vi "Update Test Server.vi"() -> ()   [LabVIEW 2013, in "OPC UA tests.lvlib"]
doc: "Forces the server to update every line in given input."
uses:
  OPC UA tests.lvlib
  <vilib>/opcua/NI OPC UA Server.lvlib
  <vilib>/OPCUA/server/Write Bool.vi
  module/configuration/OPC UA Data Type.ctl
  module/configuration/OPC UA configuration.lvclass
panel:
  out "error out":errorcluster
  in  "error in (no error)":errorcluster
  in  "OPC UA server refnum in":refnum<k21>
  in  "Items":cluster{"name":string, "OPC UA Data Type":T1}[](array[cluster])
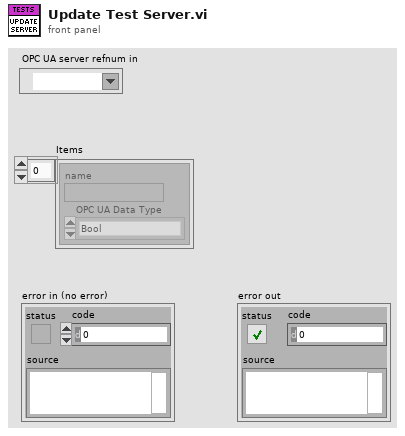
[diagram p1: front panel]
types:
  T1 = typedef "OPC UA configuration.lvclass/OPC UA Data Type.ctl" = enum16{"Bool", "SByte", "Byte", "Int16", "UInt16", "Int32", "UInt32", "Int64", "UInt64", "Float", "Double", "String", "DateTime", "ByteString", "Bool Array", "SByte Array", "Byte Array", "Int16 Array", "UInt16 Array", "Int32 Array", "UInt32 Array", "Int64 Array", "UInt64 Array", "Float Array", "Double Array", "String Array", "DateTime Array", "ByteString Array"}
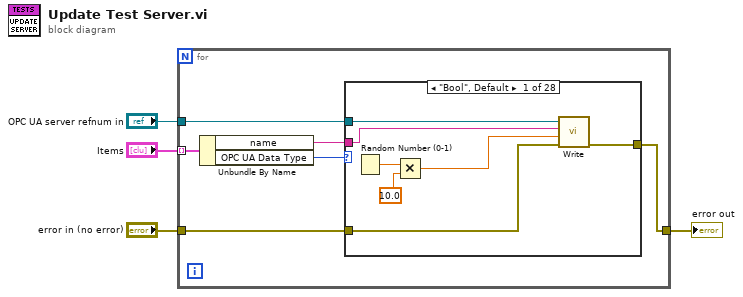
[diagram p0: block diagram]
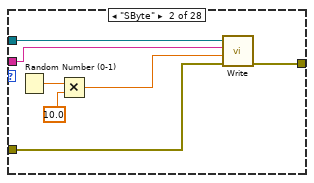
[diagram p2: hidden frame]
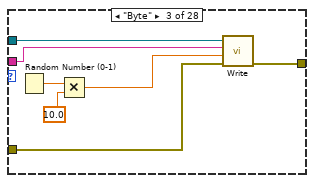
[diagram p3: hidden frame]
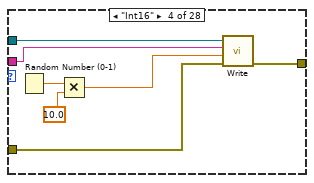
[diagram p4: hidden frame]
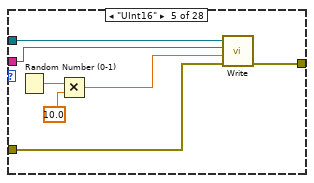
[diagram p5: hidden frame]
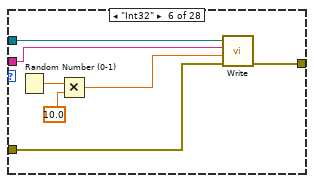
[diagram p6: hidden frame]
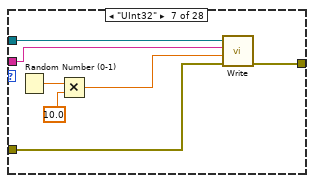
[diagram p7: hidden frame]
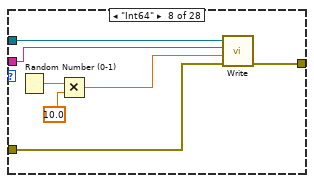
[diagram p8: hidden frame]
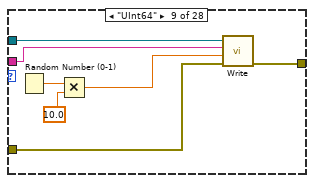
[diagram p9: hidden frame]
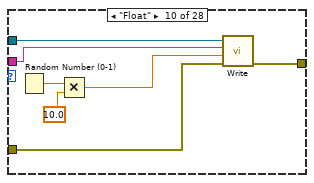
[diagram p10: hidden frame]
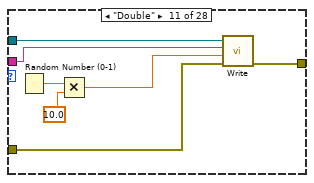
[diagram p11: hidden frame]
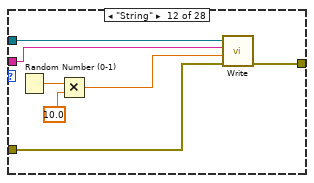
[diagram p12: hidden frame]
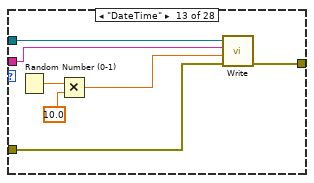
[diagram p13: hidden frame]
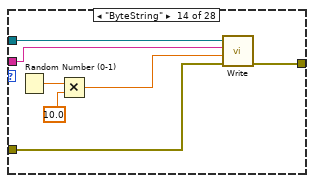
[diagram p14: hidden frame]
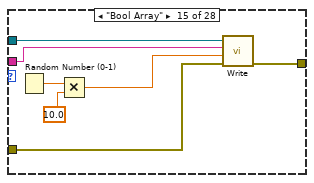
[diagram p15: hidden frame]
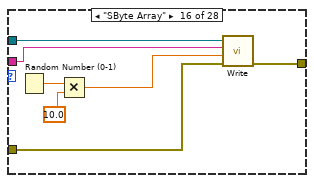
[diagram p16: hidden frame]
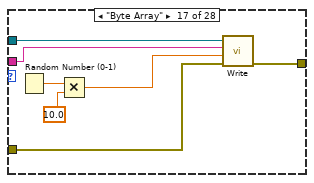
[diagram p17: hidden frame]
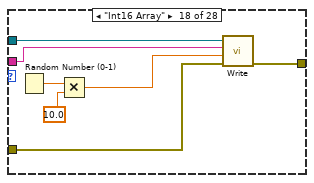
[diagram p18: hidden frame]
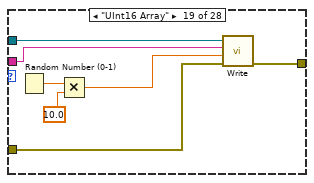
[diagram p19: hidden frame]
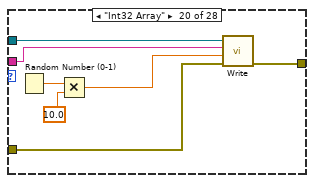
[diagram p20: hidden frame]
diagram:
  n1 = for {
    tunnel: "OPC UA server refnum in" -> [w10]
    tunnel: "Items" -> [w9] mode=indexing
    tunnel: "error in (no error)" -> [w6]
    tunnel: [w5] -> w1
    n2 = Unbundle By Name(w9) -> ("name"=w7:string, "OPC UA Data Type"=w8:T1)
    n3 = case shown="\"Bool\", Default" w8 {
      tunnel: w10 -> [w17 w24 w31 w38 w45 w52 w59 w66 w73 w80 w87 w94 w101 w108 w115 w122 w129 w136 w143 w150 w157 w164 w171 w178 w185 w192 w199 w206]
      tunnel: w7 -> [w16 w23 w30 w37 w44 w51 w58 w65 w72 w79 w86 w93 w100 w107 w114 w121 w128 w135 w142 w149 w156 w163 w170 w177 w184 w191 w198 w205]
      tunnel: w6 -> [w15 w22 w29 w36 w43 w50 w57 w64 w71 w78 w85 w92 w99 w106 w113 w120 w127 w134 w141 w148 w155 w162 w169 w176 w183 w190 w197 w204]
      tunnel: [w14 w21 w28 w35 w42 w49 w56 w63 w70 w77 w84 w91 w98 w105 w112 w119 w126 w133 w140 w147 w154 w161 w168 w175 w182 w189 w196 w203] -> w5
      frame "Bool", Default {
        n4 = Random Number (0-1)() -> (number: 0 to 1=w13:dbl)
        n5 = Multiply(x=w13, y=10.0) -> (x*y=w11:dbl)
        n6 = call-poly <vilib>:"Write.vi"("error in (no error)"=w15, "value"=w11, "node path"=w16, "OPC UA server refnum in"=w17) -> ("error out"=w14:errorcluster)  [unwired: 6 in, 1 out]
      }
      frame "SByte" {
        n7 = Random Number (0-1)() -> (number: 0 to 1=w20:dbl)
        n8 = Multiply(x=w20, y=10.0) -> (x*y=w18:dbl)
        n9 = call-poly <vilib>:"Write.vi"("error in (no error)"=w22, "value"=w18, "node path"=w23, "OPC UA server refnum in"=w24) -> ("error out"=w21:errorcluster)  [unwired: 6 in, 1 out]
      }
      frame "Byte" {
        n10 = Random Number (0-1)() -> (number: 0 to 1=w27:dbl)
        n11 = Multiply(x=w27, y=10.0) -> (x*y=w25:dbl)
        n12 = call-poly <vilib>:"Write.vi"("error in (no error)"=w29, "value"=w25, "node path"=w30, "OPC UA server refnum in"=w31) -> ("error out"=w28:errorcluster)  [unwired: 6 in, 1 out]
      }
      frame "Int16" {
        n13 = Random Number (0-1)() -> (number: 0 to 1=w34:dbl)
        n14 = Multiply(x=w34, y=10.0) -> (x*y=w32:dbl)
        n15 = call-poly <vilib>:"Write.vi"("error in (no error)"=w36, "value"=w32, "node path"=w37, "OPC UA server refnum in"=w38) -> ("error out"=w35:errorcluster)  [unwired: 6 in, 1 out]
      }
      frame "UInt16" {
        n16 = Random Number (0-1)() -> (number: 0 to 1=w41:dbl)
        n17 = Multiply(x=w41, y=10.0) -> (x*y=w39:dbl)
        n18 = call-poly <vilib>:"Write.vi"("error in (no error)"=w43, "value"=w39, "node path"=w44, "OPC UA server refnum in"=w45) -> ("error out"=w42:errorcluster)  [unwired: 6 in, 1 out]
      }
      frame "Int32" {
        n19 = Random Number (0-1)() -> (number: 0 to 1=w48:dbl)
        n20 = Multiply(x=w48, y=10.0) -> (x*y=w46:dbl)
        n21 = call-poly <vilib>:"Write.vi"("error in (no error)"=w50, "value"=w46, "node path"=w51, "OPC UA server refnum in"=w52) -> ("error out"=w49:errorcluster)  [unwired: 6 in, 1 out]
      }
      frame "UInt32" {
        n22 = Random Number (0-1)() -> (number: 0 to 1=w55:dbl)
        n23 = Multiply(x=w55, y=10.0) -> (x*y=w53:dbl)
        n24 = call-poly <vilib>:"Write.vi"("error in (no error)"=w57, "value"=w53, "node path"=w58, "OPC UA server refnum in"=w59) -> ("error out"=w56:errorcluster)  [unwired: 6 in, 1 out]
      }
      frame "Int64" {
        n25 = Random Number (0-1)() -> (number: 0 to 1=w62:dbl)
        n26 = Multiply(x=w62, y=10.0) -> (x*y=w60:dbl)
        n27 = call-poly <vilib>:"Write.vi"("error in (no error)"=w64, "value"=w60, "node path"=w65, "OPC UA server refnum in"=w66) -> ("error out"=w63:errorcluster)  [unwired: 6 in, 1 out]
      }
      frame "UInt64" {
        n28 = Random Number (0-1)() -> (number: 0 to 1=w69:dbl)
        n29 = Multiply(x=w69, y=10.0) -> (x*y=w67:dbl)
        n30 = call-poly <vilib>:"Write.vi"("error in (no error)"=w71, "value"=w67, "node path"=w72, "OPC UA server refnum in"=w73) -> ("error out"=w70:errorcluster)  [unwired: 6 in, 1 out]
      }
      frame "Float" {
        n31 = Random Number (0-1)() -> (number: 0 to 1=w76:dbl)
        n32 = Multiply(x=w76, y=10.0) -> (x*y=w74:dbl)
        n33 = call-poly <vilib>:"Write.vi"("error in (no error)"=w78, "value"=w74, "node path"=w79, "OPC UA server refnum in"=w80) -> ("error out"=w77:errorcluster)  [unwired: 6 in, 1 out]
      }
      frame "Double" {
        n34 = Random Number (0-1)() -> (number: 0 to 1=w83:dbl)
        n35 = Multiply(x=w83, y=10.0) -> (x*y=w81:dbl)
        n36 = call-poly <vilib>:"Write.vi"("error in (no error)"=w85, "value"=w81, "node path"=w86, "OPC UA server refnum in"=w87) -> ("error out"=w84:errorcluster)  [unwired: 6 in, 1 out]
      }
      frame "String" {
        n37 = Random Number (0-1)() -> (number: 0 to 1=w90:dbl)
        n38 = Multiply(x=w90, y=10.0) -> (x*y=w88:dbl)
        n39 = call-poly <vilib>:"Write.vi"("error in (no error)"=w92, "value"=w88, "node path"=w93, "OPC UA server refnum in"=w94) -> ("error out"=w91:errorcluster)  [unwired: 6 in, 1 out]
      }
      frame "DateTime" {
        n40 = Random Number (0-1)() -> (number: 0 to 1=w97:dbl)
        n41 = Multiply(x=w97, y=10.0) -> (x*y=w95:dbl)
        n42 = call-poly <vilib>:"Write.vi"("error in (no error)"=w99, "value"=w95, "node path"=w100, "OPC UA server refnum in"=w101) -> ("error out"=w98:errorcluster)  [unwired: 6 in, 1 out]
      }
      frame "ByteString" {
        n43 = Random Number (0-1)() -> (number: 0 to 1=w104:dbl)
        n44 = Multiply(x=w104, y=10.0) -> (x*y=w102:dbl)
        n45 = call-poly <vilib>:"Write.vi"("error in (no error)"=w106, "value"=w102, "node path"=w107, "OPC UA server refnum in"=w108) -> ("error out"=w105:errorcluster)  [unwired: 6 in, 1 out]
      }
      frame "Bool Array" {
        n46 = Random Number (0-1)() -> (number: 0 to 1=w111:dbl)
        n47 = Multiply(x=w111, y=10.0) -> (x*y=w109:dbl)
        n48 = call-poly <vilib>:"Write.vi"("error in (no error)"=w113, "value"=w109, "node path"=w114, "OPC UA server refnum in"=w115) -> ("error out"=w112:errorcluster)  [unwired: 6 in, 1 out]
      }
      frame "SByte Array" {
        n49 = Random Number (0-1)() -> (number: 0 to 1=w118:dbl)
        n50 = Multiply(x=w118, y=10.0) -> (x*y=w116:dbl)
        n51 = call-poly <vilib>:"Write.vi"("error in (no error)"=w120, "value"=w116, "node path"=w121, "OPC UA server refnum in"=w122) -> ("error out"=w119:errorcluster)  [unwired: 6 in, 1 out]
      }
      frame "Byte Array" {
        n52 = Random Number (0-1)() -> (number: 0 to 1=w125:dbl)
        n53 = Multiply(x=w125, y=10.0) -> (x*y=w123:dbl)
        n54 = call-poly <vilib>:"Write.vi"("error in (no error)"=w127, "value"=w123, "node path"=w128, "OPC UA server refnum in"=w129) -> ("error out"=w126:errorcluster)  [unwired: 6 in, 1 out]
      }
      frame "Int16 Array" {
        n55 = Random Number (0-1)() -> (number: 0 to 1=w132:dbl)
        n56 = Multiply(x=w132, y=10.0) -> (x*y=w130:dbl)
        n57 = call-poly <vilib>:"Write.vi"("error in (no error)"=w134, "value"=w130, "node path"=w135, "OPC UA server refnum in"=w136) -> ("error out"=w133:errorcluster)  [unwired: 6 in, 1 out]
      }
      frame "UInt16 Array" {
        n58 = Random Number (0-1)() -> (number: 0 to 1=w139:dbl)
        n59 = Multiply(x=w139, y=10.0) -> (x*y=w137:dbl)
        n60 = call-poly <vilib>:"Write.vi"("error in (no error)"=w141, "value"=w137, "node path"=w142, "OPC UA server refnum in"=w143) -> ("error out"=w140:errorcluster)  [unwired: 6 in, 1 out]
      }
      frame "Int32 Array" {
        n61 = Random Number (0-1)() -> (number: 0 to 1=w146:dbl)
        n62 = Multiply(x=w146, y=10.0) -> (x*y=w144:dbl)
        n63 = call-poly <vilib>:"Write.vi"("error in (no error)"=w148, "value"=w144, "node path"=w149, "OPC UA server refnum in"=w150) -> ("error out"=w147:errorcluster)  [unwired: 6 in, 1 out]
      }
      frame "UInt32 Array" {
        n64 = Random Number (0-1)() -> (number: 0 to 1=w153:dbl)
        n65 = Multiply(x=w153, y=10.0) -> (x*y=w151:dbl)
        n66 = call-poly <vilib>:"Write.vi"("error in (no error)"=w155, "value"=w151, "node path"=w156, "OPC UA server refnum in"=w157) -> ("error out"=w154:errorcluster)  [unwired: 6 in, 1 out]
      }
      frame "Int64 Array" {
        n67 = Random Number (0-1)() -> (number: 0 to 1=w160:dbl)
        n68 = Multiply(x=w160, y=10.0) -> (x*y=w158:dbl)
        n69 = call-poly <vilib>:"Write.vi"("error in (no error)"=w162, "value"=w158, "node path"=w163, "OPC UA server refnum in"=w164) -> ("error out"=w161:errorcluster)  [unwired: 6 in, 1 out]
      }
      frame "UInt64 Array" {
        n70 = Random Number (0-1)() -> (number: 0 to 1=w167:dbl)
        n71 = Multiply(x=w167, y=10.0) -> (x*y=w165:dbl)
        n72 = call-poly <vilib>:"Write.vi"("error in (no error)"=w169, "value"=w165, "node path"=w170, "OPC UA server refnum in"=w171) -> ("error out"=w168:errorcluster)  [unwired: 6 in, 1 out]
      }
      frame "Float Array" {
        n73 = Random Number (0-1)() -> (number: 0 to 1=w174:dbl)
        n74 = Multiply(x=w174, y=10.0) -> (x*y=w172:dbl)
        n75 = call-poly <vilib>:"Write.vi"("error in (no error)"=w176, "value"=w172, "node path"=w177, "OPC UA server refnum in"=w178) -> ("error out"=w175:errorcluster)  [unwired: 6 in, 1 out]
      }
      frame "Double Array" {
        n76 = Random Number (0-1)() -> (number: 0 to 1=w181:dbl)
        n77 = Multiply(x=w181, y=10.0) -> (x*y=w179:dbl)
        n78 = call-poly <vilib>:"Write.vi"("error in (no error)"=w183, "value"=w179, "node path"=w184, "OPC UA server refnum in"=w185) -> ("error out"=w182:errorcluster)  [unwired: 6 in, 1 out]
      }
      frame "String Array" {
        n79 = Random Number (0-1)() -> (number: 0 to 1=w188:dbl)
        n80 = Multiply(x=w188, y=10.0) -> (x*y=w186:dbl)
        n81 = call-poly <vilib>:"Write.vi"("error in (no error)"=w190, "value"=w186, "node path"=w191, "OPC UA server refnum in"=w192) -> ("error out"=w189:errorcluster)  [unwired: 6 in, 1 out]
      }
      frame "DateTime Array" {
        n82 = Random Number (0-1)() -> (number: 0 to 1=w195:dbl)
        n83 = Multiply(x=w195, y=10.0) -> (x*y=w193:dbl)
        n84 = call-poly <vilib>:"Write.vi"("error in (no error)"=w197, "value"=w193, "node path"=w198, "OPC UA server refnum in"=w199) -> ("error out"=w196:errorcluster)  [unwired: 6 in, 1 out]
      }
      frame "ByteString Array" {
        n85 = Random Number (0-1)() -> (number: 0 to 1=w202:dbl)
        n86 = Multiply(x=w202, y=10.0) -> (x*y=w200:dbl)
        n87 = call-poly <vilib>:"Write.vi"("error in (no error)"=w204, "value"=w200, "node path"=w205, "OPC UA server refnum in"=w206) -> ("error out"=w203:errorcluster)  [unwired: 6 in, 1 out]
      }
    }
  }
  "error out" <- w1
